vi "Lab Panel V5.25.vi"() -> ()   [LabVIEW 2017] (continued)
                n1783 = property on="SET LAB03-1" class="Clust (strict)"("DisabledEnum"=w3332) -> ()  [unwired: 2 in, 2 out]
                n1784 = property on="O/I  LAB01-1" class="Bool (strict)"("DisabledEnum"=w3336) -> ()  [unwired: 2 in, 2 out]
                n1785 = property on="O/I  LAB01-2" class="Bool (strict)"("DisabledEnum"=w3335) -> ()  [unwired: 2 in, 2 out]
                n1786 = property on="O/I  LAB02-1" class="Bool (strict)"("DisabledEnum"=w3334) -> ()  [unwired: 2 in, 2 out]
                n1787 = property on="O/I  LAB02-2" class="Bool (strict)"("DisabledEnum"=w3333) -> ()  [unwired: 2 in, 2 out]
                n1788 = property on="O/I  LAB03-1" class="Bool (strict)"("DisabledEnum"=w3332) -> ()  [unwired: 2 in, 2 out]
              }
              frame #1 {
                n1789 = Select(t=2, s=w3366, f=0) -> (s? t:f=w3357:i32)
                n1790 = Select(t=2, s=w3365, f=0) -> (s? t:f=w3358:i32)
                n1791 = Select(t=2, s=w3362, f=0) -> (s? t:f=w3361:i32)
                n1792 = Select(t=2, s=w3363, f=0) -> (s? t:f=w3360:i32)
                n1793 = Select(t=2, s=w3364, f=0) -> (s? t:f=w3359:i32)
                n1794 = property on="SELECT LAB05-2" class="RadioBtnsControl (strict)"("DisabledEnum"=w3357) -> ()  [unwired: 2 in, 2 out]
                n1795 = property on="SELECT LAB05-1" class="RadioBtnsControl (strict)"("DisabledEnum"=w3358) -> ()  [unwired: 2 in, 2 out]
                n1796 = property on="SELECT LAB03-2" class="RadioBtnsControl (strict)"("DisabledEnum"=w3361) -> ()  [unwired: 2 in, 2 out]
                n1797 = property on="SELECT LAB04-1" class="RadioBtnsControl (strict)"("DisabledEnum"=w3360) -> ()  [unwired: 2 in, 2 out]
                n1798 = property on="SELECT LAB04-2" class="RadioBtnsControl (strict)"("DisabledEnum"=w3359) -> ()  [unwired: 2 in, 2 out]
                n1799 = property on="SET LAB05-2" class="Clust (strict)"("DisabledEnum"=w3357) -> ()  [unwired: 2 in, 2 out]
                n1800 = property on="SET LAB05-1" class="Clust (strict)"("DisabledEnum"=w3358) -> ()  [unwired: 2 in, 2 out]
                n1801 = property on="SET LAB03-2" class="Clust (strict)"("DisabledEnum"=w3361) -> ()  [unwired: 2 in, 2 out]
                n1802 = property on="SET LAB04-1" class="Clust (strict)"("DisabledEnum"=w3360) -> ()  [unwired: 2 in, 2 out]
                n1803 = property on="SET LAB04-2" class="Clust (strict)"("DisabledEnum"=w3359) -> ()  [unwired: 2 in, 2 out]
                n1804 = property on="O/I  LAB05-2" class="Bool (strict)"("DisabledEnum"=w3357) -> ()  [unwired: 2 in, 2 out]
                n1805 = property on="O/I  LAB05-1" class="Bool (strict)"("DisabledEnum"=w3358) -> ()  [unwired: 2 in, 2 out]
                n1806 = property on="O/I  LAB04-1" class="Bool (strict)"("DisabledEnum"=w3360) -> ()  [unwired: 2 in, 2 out]
                n1807 = property on="O/I  LAB04-2" class="Bool (strict)"("DisabledEnum"=w3359) -> ()  [unwired: 2 in, 2 out]
                n1808 = property on="O/I  LAB03-2" class="Bool (strict)"("DisabledEnum"=w3361) -> ()  [unwired: 2 in, 2 out]
                n1809 = Not(x=w3366) -> (.not. x?=w3367:bool)
                n1810 = Not(x=w3365) -> (.not. x?=w3368:bool)
                n1811 = Not(x=w3364) -> (.not. x?=w3369:bool)
                n1812 = property on="RESULT LAB05-2" class="Bool (strict)"("Visible"=w3367) -> ()  [unwired: 2 in, 2 out]
                n1813 = property on="RESULT LAB05-1" class="Bool (strict)"("Visible"=w3368) -> ()  [unwired: 2 in, 2 out]
                n1814 = Not(x=w3363) -> (.not. x?=w3370:bool)
                n1815 = property on="RESULT LAB04-2" class="Bool (strict)"("Visible"=w3369) -> ()  [unwired: 2 in, 2 out]
                n1816 = Not(x=w3362) -> (.not. x?=w3371:bool)
                n1817 = property on="RESULT LAB04-1" class="Bool (strict)"("Visible"=w3370) -> ()  [unwired: 2 in, 2 out]
                n1818 = property on="RESULT LAB03-2" class="Bool (strict)"("Visible"=w3371) -> ()  [unwired: 2 in, 2 out]
              }
              frame #2 {
                # "disable calibrate if any test running"
                n1819 = Or(x=w3394, y=w3393) -> (x .or. y?=w3387:bool)
                n1820 = Or(x=w3396, y=w3395) -> (x .or. y?=w3389:bool)
                n1821 = Or(x=w3400, y=w3399) -> (x .or. y?=w3391:bool)
                n1822 = Or(x=w3398, y=w3397) -> (x .or. y?=w3390:bool)
                n1823 = Or(x=w3402, y=w3401) -> (x .or. y?=w3392:bool)
                n1824 = Or(x=w3390, y=w3389) -> (x .or. y?=w3388:bool)
                n1825 = Or(x=w3392, y=w3391) -> (x .or. y?=w3386:bool)
                n1826 = Or(x=w3388, y=w3387) -> (x .or. y?=w3385:bool)
                n1827 = Or(x=w3386, y=w3385) -> (x .or. y?=w3382:bool)
                "Any Test Running" <- w3382
                n1828 = case shown="False" w3382 {
                  tunnel: [0 2] -> w3384
                  frame False {
                  }
                  frame True {
                  }
                }
                n1829 = property on="JIG TEST" class="Clust (strict)"("DisabledEnum"=w3384) -> ()  [unwired: 2 in, 2 out]
                n1830 = property on="Network Directory" class="Path"("DisabledEnum"=w3384) -> ()  [unwired: 2 in, 2 out]
                n1831 = property on="MAIL SETTINGS" class="Clust (strict)"("DisabledEnum"=w3384) -> ()  [unwired: 2 in, 2 out]
                n1832 = property on="SET (cal)" class="Bool (strict)"("DisabledEnum"=w3384) -> ()  [unwired: 2 in, 2 out]
                n1833 = property on="ADMIN" class="Bool (strict)"("DisabledEnum"=0) -> ()  [unwired: 2 in, 2 out]
              }
            }
          }
          frame #8 {
            # "drive jigs"
            n1834 = stacked-sequence {
              frame #0 {
                # "jig on"
                n1835 = local read "jig cycle"() -> (w3410:dbl)
                n1836 = property on="JIG TEST" class="Clust (strict)"() -> ("DisabledEnum"=w3407:T16)  [unwired: 2 in, 2 out]
                n1837 = Equal?(x=w3407, y=2) -> (x = y?=w3406:bool)
                n1838 = Equal?(x=w3410, y=0) -> (x = y?=w3408:bool)
                n1839 = And(x=w3408, y=w3406) -> (x .and. y?=w3405:bool)
                n1840 = case shown="True" w3405 {
                  frame False {
                  }
                  frame True {
                    n1841 = local read "run lab01-1"() -> (w3421:bool)
                    n1842 = local read "run lab01-2"() -> (w3420:bool)
                    n1843 = local read "run lab02-1"() -> (w3419:bool)
                    n1844 = local read "run lab02-2"() -> (w3418:bool)
                    n1845 = local read "run lab03-1"() -> (w3417:bool)
                    n1846 = local read "run lab03-2"() -> (w3416:bool)
                    n1847 = local read "run lab04-1"() -> (w3415:bool)
                    n1848 = local read "run lab04-2"() -> (w3414:bool)
                    n1849 = local read "run lab05-1"() -> (w3413:bool)
                    n1850 = local read "run lab05-2"() -> (w3412:bool)
                    n1851 = local write "JIG LAB03-2"(w3416) -> ()
                    n1852 = local write "JIG LAB01-1"(w3421) -> ()
                    n1853 = local write "JIG LAB01-2"(w3420) -> ()
                    n1854 = local write "JIG LAB02-1"(w3419) -> ()
                    n1855 = local write "JIG LAB02-2"(w3418) -> ()
                    n1856 = local write "JIG LAB03-1"(w3417) -> ()
                    n1857 = local write "JIG LAB04-1"(w3415) -> ()
                    n1858 = local write "JIG LAB04-2"(w3414) -> ()
                    n1859 = local write "JIG LAB05-1"(w3413) -> ()
                    n1860 = local write "JIG LAB05-2"(w3412) -> ()
                  }
                }
              }
              frame #1 {
                # "jig off"
                n1861 = local read "jig cycle"() -> (w3428:dbl)
                n1862 = local read "on loops"() -> (w3427:dbl)
                n1863 = property on="JIG TEST" class="Clust (strict)"() -> ("DisabledEnum"=w3426:T16)  [unwired: 2 in, 2 out]
                n1864 = Equal?(x=w3426, y=2) -> (x = y?=w3424:bool)
                n1865 = Equal?(x=w3428, y=w3427) -> (x = y?=w3423:bool)
                n1866 = And(x=w3423, y=w3424) -> (x .and. y?=w3422:bool)
                n1867 = case shown="True" w3422 {
                  frame False {
                  }
                  frame True {
                    w3479 = FALSE
                    w3480 = TRUE
                    w3478 = 2
                    n1868 = local read "SELECT LAB05-2"() -> (w3469:T3)
                    n1869 = local read "SELECT LAB04-2"() -> (w3471:T3)
                    n1870 = local read "SELECT LAB04-1"() -> (w3472:T3)
                    n1871 = local read "SELECT LAB05-1"() -> (w3470:T3)
                    n1872 = local read "SELECT LAB03-2"() -> (w3473:T3)
                    n1873 = local read "SELECT LAB02-1"() -> (w3476:T3)
                    n1874 = local read "SELECT LAB03-1"() -> (w3474:T3)
                    n1875 = local read "SELECT LAB02-2"() -> (w3475:T3)
                    n1876 = local read "SELECT LAB01-2"() -> (w3477:T3)
                    n1877 = local read "run lab05-1"() -> (w3439:bool)
                    n1878 = local read "run lab05-2"() -> (w3438:bool)
                    n1879 = local read "run lab04-2"() -> (w3440:bool)
                    n1880 = local read "SELECT LAB01-1"() -> (w3481:T3)
                    n1881 = local read "run lab04-1"() -> (w3441:bool)
                    n1882 = local read "run lab01-1"() -> (w3457:bool)
                    n1883 = local read "run lab01-2"() -> (w3446:bool)
                    n1884 = local read "run lab03-2"() -> (w3442:bool)
                    n1885 = local read "run lab03-1"() -> (w3443:bool)
                    n1886 = local read "run lab02-1"() -> (w3445:bool)
                    n1887 = local read "run lab02-2"() -> (w3444:bool)
                    n1888 = Equal?(x=w3478, y=w3474) -> (x = y?=w3452:bool)
                    n1889 = Equal?(x=w3478, y=w3473) -> (x = y?=w3451:bool)
                    n1890 = Equal?(x=w3478, y=w3472) -> (x = y?=w3450:bool)
                    n1891 = Equal?(x=w3478, y=w3471) -> (x = y?=w3449:bool)
                    n1892 = Equal?(x=w3478, y=w3470) -> (x = y?=w3448:bool)
                    n1893 = Equal?(x=w3478, y=w3469) -> (x = y?=w3447:bool)
                    n1894 = Equal?(x=w3478, y=w3481) -> (x = y?=w3458:bool)
                    n1895 = Equal?(x=w3478, y=w3476) -> (x = y?=w3454:bool)
                    n1896 = Equal?(x=w3478, y=w3475) -> (x = y?=w3453:bool)
                    n1897 = Equal?(x=w3478, y=w3477) -> (x = y?=w3455:bool)
                    n1898 = And(x=w3449, y=w3440) -> (x .and. y?=w3431:bool)
                    n1899 = And(x=w3452, y=w3443) -> (x .and. y?=w3434:bool)
                    n1900 = And(x=w3450, y=w3441) -> (x .and. y?=w3432:bool)
                    n1901 = And(x=w3447, y=w3438) -> (x .and. y?=w3429:bool)
                    n1902 = And(x=w3453, y=w3444) -> (x .and. y?=w3435:bool)
                    n1903 = And(x=w3451, y=w3442) -> (x .and. y?=w3433:bool)
                    n1904 = And(x=w3448, y=w3439) -> (x .and. y?=w3430:bool)
                    n1905 = And(x=w3455, y=w3446) -> (x .and. y?=w3437:bool)
                    n1906 = And(x=w3458, y=w3457) -> (x .and. y?=w3456:bool)
                    n1907 = And(x=w3454, y=w3445) -> (x .and. y?=w3436:bool)
                    n1908 = Select(t=w3480, s=w3456, f=w3479) -> (s? t:f=w3459:bool)
                    n1909 = Select(t=w3480, s=w3437, f=w3479) -> (s? t:f=w3460:bool)
                    n1910 = Select(t=w3480, s=w3436, f=w3479) -> (s? t:f=w3461:bool)
                    n1911 = Select(t=w3480, s=w3435, f=w3479) -> (s? t:f=w3462:bool)
                    n1912 = Select(t=w3480, s=w3434, f=w3479) -> (s? t:f=w3463:bool)
                    n1913 = Select(t=w3480, s=w3433, f=w3479) -> (s? t:f=w3464:bool)
                    n1914 = Select(t=w3480, s=w3432, f=w3479) -> (s? t:f=w3465:bool)
                    n1915 = Select(t=w3480, s=w3431, f=w3479) -> (s? t:f=w3466:bool)
                    n1916 = Select(t=w3480, s=w3430, f=w3479) -> (s? t:f=w3467:bool)
                    n1917 = Select(t=w3480, s=w3429, f=w3479) -> (s? t:f=w3468:bool)
                    n1918 = local write "JIG LAB03-2"(w3464) -> ()
                    n1919 = local write "JIG LAB02-1"(w3461) -> ()
                    n1920 = local write "JIG LAB02-2"(w3462) -> ()
                    n1921 = local write "JIG LAB01-2"(w3460) -> ()
                    n1922 = local write "JIG LAB03-1"(w3463) -> ()
                    n1923 = local write "JIG LAB01-1"(w3459) -> ()
                    n1924 = local write "JIG LAB05-2"(w3468) -> ()
                    n1925 = local write "JIG LAB04-1"(w3465) -> ()
                    n1926 = local write "JIG LAB05-1"(w3467) -> ()
                    n1927 = local write "JIG LAB04-2"(w3466) -> ()
                  }
                }
              }
            }
          }
          frame #9 {
            # "enable  jig test output if no test busy"
            n1928 = property on="JIG TEST" class="Clust (strict)"() -> ("DisabledEnum"=w3484:T16)  [unwired: 2 in, 2 out]
            n1929 = Equal?(x=w3484, y=0) -> (x = y?=w3482:bool)
            n1930 = case shown="True" w3482 {
              frame False {
              }
              frame True {
                n1931 = local read "JIG TEST"() -> (w3495:T10)
                n1932 = Unbundle(w3495) -> ("LAB01-1"=w3494:bool, "LAB01-2"=w3493:bool, "LAB02-1"=w3492:bool, "LAB02-2"=w3491:bool, "LAB03-1"=w3490:bool, "LAB03-2"=w3489:bool, "LAB04-1"=w3488:bool, "LAB04-2"=w3487:bool, "LAB05-1"=w3486:bool, "LAB05-2"=w3485:bool)
                n1933 = local write "JIG LAB05-1"(w3486) -> ()
                n1934 = local write "JIG LAB05-2"(w3485) -> ()
                n1935 = local write "JIG LAB04-1"(w3488) -> ()
                n1936 = local write "JIG LAB04-2"(w3487) -> ()
                n1937 = local write "JIG LAB03-2"(w3489) -> ()
                n1938 = local write "JIG LAB01-1"(w3494) -> ()
                n1939 = local write "JIG LAB02-1"(w3492) -> ()
                n1940 = local write "JIG LAB03-1"(w3490) -> ()
                n1941 = local write "JIG LAB01-2"(w3493) -> ()
                n1942 = local write "JIG LAB02-2"(w3491) -> ()
              }
            }
          }
          frame #10 {
            w3496 = FALSE
            # "Drive digital output and reset USB and temperature network if required."
            n1943 = global read "Global display 3.vi" "cycle O/F"() -> (w3505:bool)
            n1944 = local read "O/I  LAB05-2"() -> (w3498:bool)
            n1945 = local read "O/I  LAB05-1"() -> (w3500:bool)
            n1946 = local read "JIG LAB05-2"() -> (w3497:bool)
            n1947 = local read "O/I  LAB04-2"() -> (w3502:bool)
            n1948 = local read "JIG LAB05-1"() -> (w3499:bool)
            n1949 = local read "JIG LAB04-2"() -> (w3501:bool)
            n1950 = local read "O/I  LAB03-1"() -> (w3516:bool)
            n1951 = local read "O/I  LAB04-1"() -> (w3512:bool)
            n1952 = local read "O/I  LAB02-1"() -> (w3520:bool)
            n1953 = local read "O/I  LAB02-2"() -> (w3518:bool)
            n1954 = local read "O/I  LAB03-2"() -> (w3514:bool)
            n1955 = local read "JIG LAB04-1"() -> (w3511:bool)
            n1956 = local read "JIG LAB03-2"() -> (w3513:bool)
            n1957 = local read "O/I  LAB01-2"() -> (w3522:bool)
            n1958 = local read "JIG LAB02-1"() -> (w3519:bool)
            n1959 = local read "JIG LAB02-2"() -> (w3517:bool)
            n1960 = local read "JIG LAB03-1"() -> (w3515:bool)
            n1961 = local read "O/I  LAB01-1"() -> (w3524:bool)
            n1962 = local read "JIG LAB01-2"() -> (w3521:bool)
            n1963 = local read "JIG LAB01-1"() -> (w3523:bool)
            n1964 = case shown="False" w3505 {
              tunnel: [w3636 FALSE] -> w3504
              frame False {
                n1965 = local read "Analog error"() -> (w3638:bool)
                n1966 = local read "Reset Measuring"() -> (w3637:bool)
                n1967 = Or(x=w3637, y=w3638) -> (x .or. y?=w3636:bool)
              }
              frame True {
              }
            }
            n1968 = Build Array(w3517, w3516, w3515, w3514, w3513, w3512, w3511) -> (w3509:bool[])
            "USB OUT 1" <- w3509
            n1969 = Build Array(w3524, w3523, w3522, w3521, w3520, w3519, w3518) -> (w3510:bool[])
            "USB OUT 0" <- w3510
            n1970 = Build Array(w3502, w3501, w3500, w3499, w3498, w3497, w3496, w3496) -> (w3508:bool[])
            "USB OUT 2" <- w3508
            n1971 = Not(x=w3505) -> (.not. x?=w3506:bool)
            n1972 = local read "Simulate"() -> (w3507:bool)
            n1973 = And(x=w3506, y=w3504) -> (x .and. y?=w3503:bool)
            n1974 = stacked-sequence {
              tunnel: w3510 -> [w3528 w3534]
              tunnel: w3509 -> [w3527 w3533]
              tunnel: w3508 -> [w3526 w3532]
              tunnel: w3507 -> [w3525 w3535]
              tunnel: w3503 -> [_ w3536]
              frame #0 {
                # "drive outputs for normal use"
                n1975 = case shown="False" w3525 {
                  tunnel: w3528 -> [w3531 _]
                  tunnel: w3527 -> [w3530 _]
                  tunnel: w3526 -> [w3529 _]
                  frame False {
                    n1976 = call "sub vi - Drive Relays All v6.vi"("Array #2"=w3529, "Array #1"=w3530, "Array #0"=w3531) -> ()  [unwired: 8 in, 1 out]
                  }
                  frame True {
                  }
                }
              }
              frame #1 {
                # "USB  reset routine"
                n1977 = case shown="True" w3536 {
                  tunnel: w3535 -> [_ w3540]
                  tunnel: w3534 -> [_ w3539]
                  tunnel: w3533 -> [_ w3538]
                  tunnel: w3532 -> [_ w3537]
                  frame False {
                  }
                  frame True {
                    n1978 = stacked-sequence {
                      seq-local: [w3542 _ _ _ _] -> [_ w3548 _ _ _]
                      tunnel: w3540 -> [_ w3552 _ _ _]
                      tunnel: w3539 -> [_ w3551 _ _ _]
                      tunnel: w3538 -> [_ w3550 _ _ _]
                      tunnel: w3537 -> [_ w3549 _ _ _]
                      frame #0 {
                        n1979 = case shown="False" "Auto Reset" {
                          tunnel: [w3545 FALSE] -> w3543
                          frame False {
                            n1980 = Two Button Dialog(message="System reset") -> (T button?=w3545:bool)  [unwired: 2 in]
                          }
                          frame True {
                          }
                        }
                        n1981 = disable-structure shown="Disabled" {
                          frame Disabled {
                            n1982 = local write "Tab Control 2"(5) -> ()
                          }
                          frame Enabled {
                          }
                        }
                        n1983 = Or(x="Auto Reset", y=w3543) -> (x .or. y?=w3542:bool)
                      }
                      frame #1 {
                        n1984 = case shown="True" w3548 {
                          tunnel: w3552 -> [_ w3558]
                          tunnel: w3551 -> [_ w3557]
                          tunnel: w3550 -> [_ w3556]
                          tunnel: w3549 -> [_ w3555]
                          frame False {
                          }
                          frame True {
                            n1985 = stacked-sequence {
                              tunnel: w3558 -> [_ w3576 _]
                              tunnel: bool[] [] -> [w3561 w3575 w3593]
                              tunnel: w3557 -> [_ _ w3592]
                              tunnel: w3556 -> [w3560 _ w3591]
                              tunnel: w3555 -> [w3559 _ w3590]
                              tunnel: 5000 -> [w3562 _ w3589]
                              frame #0 {
                                # "switch off test stations for system reset"
                                n1986 = stacked-sequence {
                                tunnel: w3562 -> [w3566 w3570 w3572]
                                tunnel: w3561 -> [w3565 w3569 w3573]
                                tunnel: w3560 -> [w3564 _ _]
                                tunnel: w3559 -> [w3563 w3568 _]
                                frame #0 {
                                # "drive 1st 7 inputs"
                                n1987 = call "sub vi - Drive Relays All v6.vi"("Array #2"=w3563, "Array #1"=w3564, "Array #0"=w3565) -> ()  [unwired: 8 in, 1 out]
                                n1988 = call "Message Display V1.vi"("Message"="Delay off LAB 01-1 to 02-1", "Delay mS"=w3566) -> ()  [unwired: 10 in]
                                }
                                frame #1 {
                                # "drive 2nd 7 inputs"
                                n1989 = call "sub vi - Drive Relays All v6.vi"("Array #2"=w3568, "Array #1"=w3569, "Array #0"=w3569) -> ()  [unwired: 8 in, 1 out]
                                n1990 = call "Message Display V1.vi"("Message"="Delay off LAB 02-2 to 04-1", "Delay mS"=w3570) -> ()  [unwired: 10 in]
                                }
                                frame #2 {
                                # "drive 3rd 7 inputs"
                                n1991 = call "sub vi - Drive Relays All v6.vi"("Array #2"=w3573, "Array #1"=w3573, "Array #0"=w3573) -> ()  [unwired: 8 in, 1 out]
                                n1992 = call "Message Display V1.vi"("Message"="Delay off LAB 04-2 to 05-2", "Delay mS"=w3572) -> ()  [unwired: 10 in]
                                }
                                }
                              }
                              frame #1 {
                                # "reset all usb modules"
                                n1993 = stacked-sequence {
                                tunnel: w3576 -> [_ w3580]
                                tunnel: w3575 -> [w3578 _]
                                frame #0 {
                                n1994 = call "sub vi - Drive Relays All v6.vi"("Array #2"=bool[] [FALSE, FALSE, FALSE, FALSE, FALSE, FALSE, TRUE, FALSE], "Array #1"=w3578, "Array #0"=w3578) -> ()  [unwired: 8 in, 1 out]
                                }
                                frame #1 {
                                n1995 = call "Reset Meas v 5.vi"("simulate"=w3580) -> ("Reset Error"=w3579:bool)  [unwired: 10 in]
                                n1996 = case shown="False" w3579 {
                                frame False {
                                n1997 = local read "AI Task2"() -> (w3587:dbl)
                                n1998 = local read "AI Task1"() -> (w3586:dbl)
                                n1999 = local read "AI Task0"() -> (w3585:dbl)
                                n2000 = call "sub vi - AI USB4704 (3)  Create Task v2.vi"("Task In 0"=w3585, "Task In 1"=w3586, "Task In 2"=w3587) -> ("TASK USB 0"=w3584:i32, "TASK USB 1"=w3583:i32, "TASK USB 2"=w3582:i32, "AI Task Er"=w3581:bool)  [unwired: 8 in, 1 out]
                                n2001 = local write "AI Task"(w3581) -> ()
                                n2002 = local write "AI Task2"(w3582) -> ()
                                n2003 = local write "AI Task1"(w3583) -> ()
                                n2004 = local write "AI Task0"(w3584) -> ()
                                }
                                frame True {
                                "Reset Error" <- TRUE
                                }
                                }
                                }
                                }
                              }
                              frame #2 {
                                # "switch test stations back on after reset"
                                n2005 = stacked-sequence {
                                tunnel: w3593 -> [w3597 w3600 _]
                                tunnel: w3592 -> [w3596 w3602 w3607]
                                tunnel: w3589 -> [w3595 w3598 w3604]
                                tunnel: w3591 -> [_ w3601 w3606]
                                tunnel: w3590 -> [_ _ w3603]
                                frame #0 {
                                # "drive 1st 7 inputs"
                                n2006 = call "sub vi - Drive Relays All v6.vi"("Array #2"=w3597, "Array #1"=w3597, "Array #0"=w3596) -> ()  [unwired: 8 in, 1 out]
                                n2007 = call "Message Display V1.vi"("Message"="Delay on LAB 01-1 to 02-1", "Delay mS"=w3595) -> ()  [unwired: 10 in]
                                }
                                frame #1 {
                                # "drive 1st & 2nd outputs"
                                n2008 = call "sub vi - Drive Relays All v6.vi"("Array #2"=w3600, "Array #1"=w3601, "Array #0"=w3602) -> ()  [unwired: 8 in, 1 out]
                                n2009 = call "Message Display V1.vi"("Message"="Delay on LAB 02-2 to 04-1", "Delay mS"=w3598) -> ()  [unwired: 10 in]
                                }
                                frame #2 {
                                n2010 = call "sub vi - Drive Relays All v6.vi"("Array #2"=w3603, "Array #1"=w3606, "Array #0"=w3607) -> ()  [unwired: 8 in, 1 out]
                                n2011 = call "Message Display V1.vi"("Message"="Delay on LAB 04-2 to 05-2", "Delay mS"=w3604) -> ()  [unwired: 10 in]
                                }
                                }
                              }
                            }
                          }
                        }
                      }
                      frame #2 {
                        w3608 = 0
                        w3609 = FALSE
                        # "set all back to zero"
                        n2012 = local read "Total USB resets"() -> (w3611:dbl)
                        n2013 = local read "Resets Done"() -> (w3613:dbl)
                        n2014 = local write "Reset Measuring"(w3609) -> ()
                        n2015 = local write "Analog error"(w3609) -> ()
                        n2016 = local write "Er USB#2"(w3608) -> ()
                        n2017 = local write "Er USB#0"(w3608) -> ()
                        n2018 = local write "Er USB#1"(w3608) -> ()
                        n2019 = local write "Error USB #0"(w3609) -> ()
                        n2020 = local write "Error USB #1"(w3609) -> ()
                        n2021 = local write "Error USB #2"(w3609) -> ()
                        n2022 = Increment(x=w3611) -> (x+1=w3610:dbl)
                        n2023 = Increment(x=w3613) -> (x+1=→"Resets Done":dbl)
                        n2024 = local write "Total USB resets"(w3610) -> ()
                      }
                      frame #3 {
                        # "save reset value"
                        n2025 = String To Path(string="c:\\crabtree\\Set Up\\") -> (path=w3623:path)
                        n2026 = Build Path(base path=w3623, name or relative path="USB resets.bin") -> (appended path=w3616:path)
                        n2027 = Create Folder(path (use dialog)=w3623) -> (error out=w3615:errorcluster)  [unwired: 2 in, 2 out]
                        n2028 = local read "Total USB resets"() -> (w3614:dbl)
                        n2029 = call <vilib>:"Clear Errors.vi"("error in (no error)"=w3615) -> ()  [unwired: 5 in, 2 out]
                        n2030 = Open/Create/Replace File(file path (use dialog)=w3616, operation (0:open)=T17."replace or create") -> (refnum out=w3621:refnum<file>, error out=w3620:errorcluster)  [unwired: 4 in, 1 out]
                        n2031 = Write to Binary File(file (use dialog)=w3621, data=w3614, error in=w3620) -> (refnum out=w3619:refnum<file>, error out=w3618:errorcluster)  [unwired: 3 in, 1 out]
                        n2032 = Close File(refnum=w3619, error in=w3618) -> (error out=w3617:errorcluster)  [unwired: 1 out]
                        n2033 = local write "data file error"(w3617) -> ()
                      }
                      frame #4 {
                        # "mail reset value"
                        n2034 = local read "Total USB resets"() -> (w3632:dbl)
                        n2035 = local read "MAIL SETTINGS"() -> (w3628:T7)
                        n2036 = local read "Mail Test File To:"() -> (w3633:string)
                        n2037 = Number To Decimal String(number=w3632) -> (decimal integer string=w3630:string)  [unwired: 1 in]
                        n2038 = Unbundle(w3628) -> ("OUT SERVER ADDRESS"=w3635:string, "FROM ACCOUNT"=w3634:string)  [unwired: 5 out]
                        n2039 = Concatenate Strings("Total USB resets: ", w3630) -> (w3629:string)
                        n2040 = call "Lab Send Mail Test.vi"("TO:"=w3633, "subject"=w3629, "from"=w3634, "out going server"=w3635) -> ("error out"=w3627:errorcluster)  [unwired: 11 in]
                        n2041 = Bundle(cluster=w3628, "mail error"=w3627) -> (w3626:T7)  [unwired: 6 in]
                        n2042 = local write "MAIL SETTINGS"(w3626) -> ()
                      }
                    }
                  }
                }
              }
            }
          }
          frame #11 {
            # "if all test panels are off stop analog read"
            n2043 = local read "O/I  LAB03-1"() -> (w3656:bool)
            n2044 = local read "O/I  LAB03-2"() -> (w3655:bool)
            n2045 = local read "O/I  LAB04-1"() -> (w3654:bool)
            n2046 = local read "O/I  LAB04-2"() -> (w3653:bool)
            n2047 = local read "O/I  LAB05-1"() -> (w3652:bool)
            n2048 = local read "O/I  LAB05-2"() -> (w3651:bool)
            n2049 = local read "O/I  LAB02-2"() -> (w3657:bool)
            n2050 = local read "O/I  LAB02-1"() -> (w3658:bool)
            n2051 = local read "O/I  LAB01-2"() -> (w3659:bool)
            n2052 = local read "O/I  LAB01-1"() -> (w3660:bool)
            n2053 = Or(x=w3652, y=w3651) -> (x .or. y?=w3649:bool)
            n2054 = Or(x=w3654, y=w3653) -> (x .or. y?=w3650:bool)
            n2055 = Or(x=w3658, y=w3657) -> (x .or. y?=w3648:bool)
            n2056 = Or(x=w3656, y=w3655) -> (x .or. y?=w3646:bool)
            n2057 = Or(x=w3660, y=w3659) -> (x .or. y?=w3647:bool)
            n2058 = Or(x=w3650, y=w3649) -> (x .or. y?=w3643:bool)
            n2059 = Or(x=w3647, y=w3648) -> (x .or. y?=w3645:bool)
            n2060 = Or(x=w3645, y=w3646) -> (x .or. y?=w3644:bool)
            n2061 = local read "Any Test Running"() -> (w3642:bool)
            n2062 = Or(x=w3644, y=w3643) -> (x .or. y?=w3641:bool)
            n2063 = Or(x=w3641, y=w3642) -> (x .or. y?=w3640:bool)
          }
          frame #12 {
            # "get all analog values from USB devices"
            n2064 = local read "on loops"() -> (w3668:dbl)
            n2065 = local read "jig cycle"() -> (w3665:dbl)
            n2066 = Add(x=w3668, y=1) -> (x+y=w3666:dbl)
            n2067 = Equal?(x=w3665, y=1) -> (x = y?=w3663:bool)
            n2068 = Equal?(x=w3665, y=w3666) -> (x = y?=w3664:bool)
            n2069 = Or(x=w3663, y=w3664) -> (x .or. y?=w3662:bool)
            n2070 = global write "Global display 3.vi" "cycle O/F"(w3663) -> ()
            n2071 = case shown="True" w3662 {
              tunnel: w3663 -> [_ w3673]
              tunnel: w3661 -> [_ w3670]
              frame False {
              }
              frame True {
                n2072 = local read "Simulate"() -> (w3676:bool)
                n2073 = case shown="False" w3676 {
                  tunnel: [w3693 0.3 ("Analog loop time")] -> w3683
                  tunnel: [w3692 dynamicdata[] [] ("array GRAPH")] -> w3682
                  tunnel: [w3691 w3716] -> w3681
                  tunnel: [w3690 w3716] -> w3680
                  tunnel: [w3689 w3716] -> w3679
                  tunnel: [w3688 w3716] -> w3678
                  tunnel: [w3687 w3716] -> w3677
                  tunnel: w3673 -> [_ w3720]
                  tunnel: [w3686 "Ambient Volts"] -> w3672
                  tunnel: [w3685 bool[] []] -> w3671
                  tunnel: w3670 -> [w3684 _]
                  frame False {
                    # "analog in"
                    n2074 = case shown="True" w3684 {
                      tunnel: [0 w3711] -> w3693
                      tunnel: [dynamicdata[] [] ("array GRAPH") w3710] -> w3692
                      tunnel: [w3694 w3709] -> w3691
                      tunnel: [w3694 w3708] -> w3690
                      tunnel: [w3694 w3707] -> w3689
                      tunnel: [w3694 w3706] -> w3688
                      tunnel: [w3694 w3705] -> w3687
                      tunnel: [3 w3704] -> w3686
                      tunnel: [bool[] [] w3703] -> w3685
                      frame False {
                        w3695 = 0.0
                        # "no test"
                        n2075 = Bundle(w3695, w3695, w3695, w3695, w3695, w3695) -> (w3694:cluster{dbl, dbl, dbl, dbl, dbl, dbl})  [unwired: 1 in]
                      }
                      frame True {
                        # "test on"
                        n2076 = local read "AI Task2"() -> (w3701:dbl)
                        n2077 = local read "AI Task1"() -> (w3700:dbl)
                        n2078 = local read "AI Task0"() -> (w3702:dbl)
                        n2079 = call "sub vi - Read Analog All v9.3.vi"("AI Task0"=w3702, "AI Task1"=w3700, "AI Task2"=w3701) -> ("Analog loop time"=w3711:dbl, "array GRAPH"=w3710:dynamicdata[], "LAB01"=w3709:T27, "LAB02"=w3708:T28, "LAB03"=w3707:T29, "LAB04"=w3706:T30, "deg C"=w3704:dbl, "USB Error"=w3703:bool[], "LAB05"=w3705:T31)  [unwired: 4 in]
                      }
                    }
                  }
                  frame True {
                    # "simulate"
                    n2080 = local read "ON amps"() -> (w3714:dbl)
                    n2081 = local read "OFF amps"() -> (w3715:dbl)
                    n2082 = local read "VOLTS"() -> (w3718:dbl)
                    n2083 = local read "PF"() -> (w3717:dbl)
                    n2084 = Select(t=w3714, s=w3720, f=w3715) -> (s? t:f=w3719:dbl)
                    n2085 = Bundle("OFF amps"=w3719, "VOLTS"=w3718, "PF"=w3717, "OFF amps"=w3719, "VOLTS"=w3718, "PF"=w3717) -> (w3716:T32)  [unwired: 1 in]
                  }
                }
                n2086 = local read "Simulate"() -> (w3675:bool)
                n2087 = stacked-sequence {
                  seq-local: [w3725 _ _ _ _ _ _ _] -> [_ _ _ _ _ _ _ _]
                  seq-local: [w3724 _ _ _ _ _ _ _] -> [_ _ _ _ _ _ _ _]
                  seq-local: [w3723 _ _ _ _ _ _ _] -> [_ _ _ _ _ _ _ w3920]
                  tunnel: w3683 -> [_ w3778 _ _ _ _ _ _]
                  tunnel: w3682 -> [_ w3775 _ _ _ _ _ _]
                  tunnel: w3681 -> [_ _ w3805 _ _ _ _ _]
                  tunnel: w3680 -> [_ _ _ w3833 _ _ _ _]
                  tunnel: w3679 -> [_ _ _ _ w3861 _ _ _]
                  tunnel: w3678 -> [_ _ _ _ _ w3889 _ _]
                  tunnel: w3677 -> [_ _ _ _ _ _ w3917 _]
                  tunnel: w3675 -> [_ _ w3804 w3832 w3860 w3888 w3916 w3922]
                  tunnel: T14 {"1  (A) cal"=1.0, "1 (V) cal"=1.0, "1 (PF) cal"=1.0, "1 (TL) cal"=1.0, "1 (TN) cal"=1.0, "2 (A) cal"=1.0, "2 (V) cal"=1.0, "2 (PF) cal"=1.0, "2 (TL) cal"=1.0, "2 (TN) cal"=1.0} ("CAL LAB01") -> [_ _ w3803 w3831 w3859 w3887 w3915 _]
                  tunnel: w3672 -> [_ _ _ _ _ _ _ w3921]
                  tunnel: w3671 -> [w3728 _ _ _ _ _ _ _]
                  frame #0 {
                    n2088 = Index Array(array=w3728, index=2) -> (element=w3723:bool)
                    n2089 = Index Array(array=w3728, index=1) -> (element=w3724:bool)
                    n2090 = Index Array(array=w3728, index=0) -> (element=w3725:bool)
                    n2091 = local write "Error USB #2"(w3723) -> ()
                    n2092 = local write "Error USB #0"(w3725) -> ()
                    n2093 = local write "Error USB #1"(w3724) -> ()
                    n2094 = stacked-sequence {
                      tunnel: w3725 -> [w3732 _ _ _]
                      tunnel: w3724 -> [_ w3737 _ _]
                      tunnel: 0 -> [w3731 w3736 w3741 _]
                      tunnel: w3723 -> [_ _ w3742 _]
                      frame #0 {
                        n2095 = case shown="True" w3732 {
                          tunnel: w3731 -> [w3733 _]
                          frame False {
                            n2096 = local write "Er USB#0"(w3733) -> ()
                          }
                          frame True {
                            n2097 = local read "Er USB#0"() -> (w3735:dbl)
                            n2098 = Increment(x=w3735) -> (x+1=→"Er USB#0":dbl)
                          }
                        }
                      }
                      frame #1 {
                        n2099 = case shown="True" w3737 {
                          tunnel: w3736 -> [w3738 _]
                          frame False {
                            n2100 = local write "Er USB#1"(w3738) -> ()
                          }
                          frame True {
                            n2101 = local read "Er USB#1"() -> (w3740:dbl)
                            n2102 = Increment(x=w3740) -> (x+1=→"Er USB#1":dbl)
                          }
                        }
                      }
                      frame #2 {
                        n2103 = case shown="True" w3742 {
                          tunnel: w3741 -> [w3743 _]
                          frame False {
                            n2104 = local write "Er USB#2"(w3743) -> ()
                          }
                          frame True {
                            n2105 = local read "Er USB#2"() -> (w3745:dbl)
                            n2106 = Increment(x=w3745) -> (x+1=→"Er USB#2":dbl)
                          }
                        }
                      }
                      frame #3 {
                        w3751 = 5
                        n2107 = local read "Er USB#2"() -> (w3752:dbl)
                        n2108 = local read "Er USB#0"() -> (w3754:dbl)
                        n2109 = local read "Er USB#1"() -> (w3753:dbl)
                        n2110 = Greater Or Equal?(x=w3754, y=w3751) -> (x >= y?=w3749:bool)
                        n2111 = Greater Or Equal?(x=w3753, y=w3751) -> (x >= y?=w3748:bool)
                        n2112 = Greater Or Equal?(x=w3752, y=w3751) -> (x >= y?=w3747:bool)
                        n2113 = Or(x=w3749, y=w3748) -> (x .or. y?=w3750:bool)
                        n2114 = Or(x=w3750, y=w3747) -> (x .or. y?=→"Analog error":bool)
                      }
                    }
                  }
                  frame #1 {
                    # "display graph data on ADM page"
                    n2115 = local write "AI"(TRUE) -> ()
                    n2116 = global write "Global 1.vi" "RATE(Hz)"("RATE (Hz)") -> ()
                    n2117 = global write "Global 1.vi" "SAMPLES"("SAMPLES") -> ()
                    n2118 = Index Array(array=w3775, index=6) -> (element=→"LAB04-1 (GRAPH)":dynamicdata)
                    n2119 = Index Array(array=w3775, index=7) -> (element=→"LAB04-2 (GRAPH)":dynamicdata)
                    n2120 = Index Array(array=w3775, index=9) -> (element=→"LAB05-2 (GRAPH)":dynamicdata)
                    n2121 = Index Array(array=w3775, index=8) -> (element=→"LAB05-1 (GRAPH)":dynamicdata)
                    n2122 = Index Array(array=w3775, index=5) -> (element=→"LAB03-2 (GRAPH)":dynamicdata)
                    n2123 = Index Array(array=w3775, index=0) -> (element=→"LAB01-1 (GRAPH)":dynamicdata)
                    n2124 = Index Array(array=w3775, index=1) -> (element=→"LAB01-2 (GRAPH)":dynamicdata)
                    n2125 = Index Array(array=w3775, index=2) -> (element=→"LAB02-1 (GRAPH)":dynamicdata)
                    n2126 = Index Array(array=w3775, index=3) -> (element=→"LAB02-2 (GRAPH)":dynamicdata)
                    n2127 = Index Array(array=w3775, index=4) -> (element=→"LAB03-1 (GRAPH)":dynamicdata)
                    "AI loop time" <- w3778
                  }
                  frame #2 {
                    n2128 = case shown="False" w3804 {
                      tunnel: [w3806 w3807] -> w3802
                      tunnel: w3803 -> [_ w3807]
                      frame False {
                        n2129 = local read "CAL LAB01"() -> (w3806:T14)
                      }
                      frame True {
                      }
                    }
                    n2130 = Unbundle By Name(w3805) -> ("OFF amps"=w3801:dbl, "VOLTS"=w3800:dbl, "PF"=w3799:dbl, "OFF amps"=w3798:dbl, "VOLTS"=w3797:dbl, "PF"=w3796:dbl)
                    n2131 = Unbundle By Name(w3802) -> ("1  (A) cal"=w3795:dbl, "1 (V) cal"=w3794:dbl, "1 (PF) cal"=w3793:dbl, "2 (A) cal"=w3792:dbl, "2 (V) cal"=w3791:dbl, "2 (PF) cal"=w3790:dbl)  [unwired: 4 out]
                    n2132 = Multiply(x=w3801, y=w3795) -> (x*y=w3788:dbl)
                    n2133 = Multiply(x=w3800, y=w3794) -> (x*y=w3787:dbl)
                    n2134 = Multiply(x=w3799, y=w3793) -> (x*y=w3786:dbl)
                    n2135 = Multiply(x=w3798, y=w3792) -> (x*y=w3784:dbl)
                    n2136 = Multiply(x=w3797, y=w3791) -> (x*y=w3783:dbl)
                    n2137 = Multiply(x=w3796, y=w3790) -> (x*y=w3782:dbl)
                    n2138 = local read "SIG LAB01-1"() -> (w3789:T2)
                    n2139 = local read "SIG LAB01-2"() -> (w3785:T2)
                    n2140 = Bundle By Name(cluster=w3789, "AMPS"=w3788, "VOLTS"=w3787, "PF"=w3786) -> (w3781:T2)
                    n2141 = Bundle By Name(cluster=w3785, "AMPS"=w3784, "VOLTS"=w3783, "PF"=w3782) -> (w3780:T2)
                    n2142 = global write "Global display 1.vi" "SIG LAB01-2"(w3780) -> ()
                    n2143 = global write "Global display 1.vi" "SIG LAB01-1"(w3781) -> ()
                    n2144 = local write "SIG LAB01-2"(w3780) -> ()
                    n2145 = local write "SIG LAB01-1"(w3781) -> ()
                  }
                  frame #3 {
                    n2146 = Unbundle By Name(w3833) -> ("OFF amps"=w3829:dbl, "VOLTS"=w3828:dbl, "PF"=w3827:dbl, "OFF amps"=w3826:dbl, "VOLTS"=w3825:dbl, "PF"=w3824:dbl)
                    n2147 = case shown="True" w3832 {
                      tunnel: [w3834 w3835] -> w3830
                      tunnel: w3831 -> [_ w3835]
                      frame False {
                        n2148 = local read "CAL LAB02"() -> (w3834:T15)
                      }
                      frame True {
                      }
                    }
                    n2149 = Unbundle By Name(w3830) -> ("1  (A) cal"=w3823:dbl, "1 (V) cal"=w3822:dbl, "1 (PF) cal"=w3821:dbl, "2 (A) cal"=w3820:dbl, "2 (V) cal"=w3819:dbl, "2 (PF) cal"=w3818:dbl)  [unwired: 4 out]
                    n2150 = Multiply(x=w3829, y=w3823) -> (x*y=w3816:dbl)
                    n2151 = Multiply(x=w3828, y=w3822) -> (x*y=w3815:dbl)
                    n2152 = Multiply(x=w3827, y=w3821) -> (x*y=w3814:dbl)
                    n2153 = Multiply(x=w3826, y=w3820) -> (x*y=w3812:dbl)
                    n2154 = Multiply(x=w3825, y=w3819) -> (x*y=w3811:dbl)
                    n2155 = Multiply(x=w3824, y=w3818) -> (x*y=w3810:dbl)
                    n2156 = local read "SIG LAB02-1"() -> (w3817:T2)
                    n2157 = local read "SIG LAB02-2"() -> (w3813:T2)
                    n2158 = Bundle By Name(cluster=w3817, "AMPS"=w3816, "VOLTS"=w3815, "PF"=w3814) -> (w3809:T2)
                    n2159 = Bundle By Name(cluster=w3813, "AMPS"=w3812, "VOLTS"=w3811, "PF"=w3810) -> (w3808:T2)
                    n2160 = global write "Global display 1.vi" "SIG LAB02-1"(w3809) -> ()
                    n2161 = local write "SIG LAB02-2"(w3808) -> ()
                    n2162 = global write "Global display 1.vi" "SIG LAB02-2"(w3808) -> ()
                    n2163 = local write "SIG LAB02-1"(w3809) -> ()
                  }
                  frame #4 {
                    n2164 = Unbundle By Name(w3861) -> ("OFF amps"=w3857:dbl, "VOLTS"=w3856:dbl, "PF"=w3855:dbl, "OFF amps"=w3854:dbl, "VOLTS"=w3853:dbl, "PF"=w3852:dbl)
                    n2165 = case shown="True" w3860 {
                      tunnel: [w3862 w3863] -> w3858
                      tunnel: w3859 -> [_ w3863]
                      frame False {
                        n2166 = local read "CAL LAB03"() -> (w3862:T14)
                      }
                      frame True {
                      }
                    }
                    n2167 = Unbundle By Name(w3858) -> ("1  (A) cal"=w3851:dbl, "1 (V) cal"=w3850:dbl, "1 (PF) cal"=w3849:dbl, "2 (A) cal"=w3848:dbl, "2 (V) cal"=w3847:dbl, "2 (PF) cal"=w3846:dbl)  [unwired: 4 out]
                    n2168 = Multiply(x=w3857, y=w3851) -> (x*y=w3844:dbl)
                    n2169 = Multiply(x=w3856, y=w3850) -> (x*y=w3838:dbl)
                    n2170 = Multiply(x=w3855, y=w3849) -> (x*y=w3843:dbl)
                    n2171 = Multiply(x=w3854, y=w3848) -> (x*y=w3841:dbl)
                    n2172 = Multiply(x=w3853, y=w3847) -> (x*y=w3840:dbl)
                    n2173 = Multiply(x=w3852, y=w3846) -> (x*y=w3839:dbl)
                    n2174 = local read "SIG LAB03-1"() -> (w3845:T2)
                    n2175 = local read "SIG LAB03-2"() -> (w3842:T2)
                    n2176 = Bundle By Name(cluster=w3845, "AMPS"=w3844, "VOLTS"=w3838, "PF"=w3843) -> (w3837:T2)
                    n2177 = Bundle By Name(cluster=w3842, "AMPS"=w3841, "VOLTS"=w3840, "PF"=w3839) -> (w3836:T2)
                    n2178 = global write "Global display 1.vi" "SIG LAB03-1"(w3837) -> ()
                    n2179 = global write "Global display 1.vi" "SIG LAB03-2"(w3836) -> ()
                    n2180 = local write "SIG LAB03-2"(w3836) -> ()
                    n2181 = local write "SIG LAB03-1"(w3837) -> ()
                  }
                  frame #5 {
                    n2182 = case shown="False" w3888 {
                      tunnel: [w3890 w3891] -> w3886
                      tunnel: w3887 -> [_ w3891]
                      frame False {
                        n2183 = local read "CAL LAB04"() -> (w3890:T14)
                      }
                      frame True {
                      }
                    }
                    n2184 = Unbundle By Name(w3889) -> ("OFF amps"=w3885:dbl, "VOLTS"=w3884:dbl, "PF"=w3883:dbl, "OFF amps"=w3882:dbl, "VOLTS"=w3881:dbl, "PF"=w3880:dbl)
                    n2185 = Unbundle By Name(w3886) -> ("1  (A) cal"=w3879:dbl, "1 (V) cal"=w3878:dbl, "1 (PF) cal"=w3877:dbl, "2 (A) cal"=w3876:dbl, "2 (V) cal"=w3875:dbl, "2 (PF) cal"=w3874:dbl)  [unwired: 4 out]
                    n2186 = Multiply(x=w3885, y=w3879) -> (x*y=w3872:dbl)
                    n2187 = Multiply(x=w3884, y=w3878) -> (x*y=w3871:dbl)
                    n2188 = Multiply(x=w3883, y=w3877) -> (x*y=w3870:dbl)
                    n2189 = Multiply(x=w3882, y=w3876) -> (x*y=w3868:dbl)
                    n2190 = Multiply(x=w3881, y=w3875) -> (x*y=w3867:dbl)
                    n2191 = Multiply(x=w3880, y=w3874) -> (x*y=w3866:dbl)
                    n2192 = local read "SIG LAB04-1"() -> (w3873:T2)
                    n2193 = local read "SIG LAB04-2"() -> (w3869:T2)
                    n2194 = Bundle By Name(cluster=w3873, "AMPS"=w3872, "VOLTS"=w3871, "PF"=w3870) -> (w3865:T2)
                    n2195 = Bundle By Name(cluster=w3869, "AMPS"=w3868, "VOLTS"=w3867, "PF"=w3866) -> (w3864:T2)
                    n2196 = global write "Global display 1.vi" "SIG LAB04-2"(w3864) -> ()
                    n2197 = global write "Global display 1.vi" "SIG LAB04-1"(w3865) -> ()
                    n2198 = local write "SIG LAB04-2"(w3864) -> ()
                    n2199 = local write "SIG LAB04-1"(w3865) -> ()
                  }
                  frame #6 {
                    n2200 = Unbundle By Name(w3917) -> ("OFF amps"=w3913:dbl, "VOLTS"=w3894:dbl, "PF"=w3912:dbl, "OFF amps"=w3911:dbl, "VOLTS"=w3910:dbl, "PF"=w3909:dbl)
                    n2201 = case shown="False" w3916 {
                      tunnel: [w3918 w3919] -> w3914
                      tunnel: w3915 -> [_ w3919]
                      frame False {
                        n2202 = local read "CAL LAB05"() -> (w3918:T14)
                      }
                      frame True {
                      }
                    }
                    n2203 = Unbundle By Name(w3914) -> ("1  (A) cal"=w3908:dbl, "1 (V) cal"=w3907:dbl, "1 (PF) cal"=w3906:dbl, "2 (A) cal"=w3905:dbl, "2 (V) cal"=w3904:dbl, "2 (PF) cal"=w3903:dbl)  [unwired: 4 out]
                    n2204 = Multiply(x=w3913, y=w3908) -> (x*y=w3901:dbl)
                    n2205 = Multiply(x=w3894, y=w3907) -> (x*y=w3900:dbl)
                    n2206 = Multiply(x=w3912, y=w3906) -> (x*y=w3899:dbl)
                    n2207 = Multiply(x=w3911, y=w3905) -> (x*y=w3897:dbl)
                    n2208 = Multiply(x=w3910, y=w3904) -> (x*y=w3896:dbl)
                    n2209 = Multiply(x=w3909, y=w3903) -> (x*y=w3895:dbl)
                    n2210 = local read "SIG LAB05-1"() -> (w3902:T2)
                    n2211 = local read "SIG LAB05-2"() -> (w3898:T2)
                    n2212 = Bundle By Name(cluster=w3902, "AMPS"=w3901, "VOLTS"=w3900, "PF"=w3899) -> (w3893:T2)
                    n2213 = Bundle By Name(cluster=w3898, "AMPS"=w3897, "VOLTS"=w3896, "PF"=w3895) -> (w3892:T2)
                    n2214 = global write "Global display 1.vi" "SIG LAB05-1"(w3893) -> ()
                    n2215 = global write "Global display 1.vi" "SIG LAB05-2"(w3892) -> ()
                    n2216 = local write "SIG LAB05-2"(w3892) -> ()
                    n2217 = local write "SIG LAB05-1"(w3893) -> ()
                  }
                  frame #7 {
                    n2218 = case shown="False" w3920 {
                      tunnel: w3922 -> [w3927 _]
                      tunnel: w3921 -> [w3926 _]
